vi "Begin.vi"(8 "error in":errorcluster) -> (0 "error out":errorcluster)   [LabVIEW 2015]
doc: "Called before other user functions, this VI is expected to open initial I/O refnums, load in file data, and do all program initialization. Notice that the <B>error out</B> terminal is simply used for data flow. Wiring it to other structures or subVIs ensures that this VI runs first."
uses:
  <vilib>/Rock Robotics/WPI/DriverStation/WPI_DriverStationRobotMode2.ctl
  Robot Global Data.vi
  <vilib>/Rock Robotics/WPI/Utilities/WPI_GetSetVariantRefNum.vi
  Library/REV Digit MXP/LabVIEW/REV Robotics Digit - Library.llb/REVDigit.lvlib
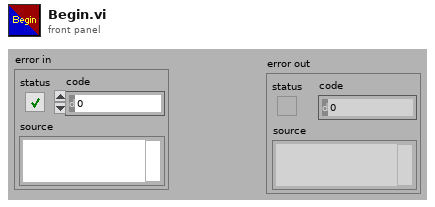
[diagram p1: front panel]
types:
  T1 = typedef "WPI_DriverStationRobotMode2.ctl" = enum16{"Autonomous Disabled", "Autonomous Enabled", "Teleop Disabled", "Teleop Enabled", "Disconnected", "Finish", "Test Disabled", "Test Enabled", "Emergency Stopped"}
  T2 = typedef "WPI_CompressorDevRef.ctl" = cluster{"DevStatus":errorcluster, "Pneumatics Control Module":u8}
  T3 = typedef "REVDigit.lvlib/REVDigitDefRef.ctl" = cluster{"HT16K33":T4, "Potentiometer":T6, "Button A":T8, "Button B":T8}
  T4 = typedef "WPI_I2CDevRef.ctl" = cluster{"DevStatus":errorcluster, "Device Address":u8, "Handle":i32, "I2C Bus":T5}
  T5 = typedef "i2c_bus.ctl" = enum16{"I2C On-Board", "I2C MXP", "Invalid"}
  T6 = typedef "WPI_AnalogChannelDevRef.ctl" = cluster{"DevStatus":errorcluster, "Analog Channel":T7}
  T7 = typedef "FPGA_AIChannel.ctl" = enum8{"AI 0", "AI 1", "AI 2", "AI 3", "AI MXP 0", "AI MXP 1", "AI MXP 2", "AI MXP 3", "Invalid"}
  T8 = typedef "WPI_DigitalInputDevRef.ctl" = cluster{"DevStatus":errorcluster, "DIO Channel":T9}
  T9 = typedef "FPGA_DIOChannel.ctl" = enum8{"DIO 0", "DIO 1", "DIO 2", "DIO 3", "DIO 4", "DIO 5", "DIO 6", "DIO 7", "DIO 8", "DIO 9", "DIO MXP 0", "DIO MXP 1", "DIO MXP 2", "DIO MXP 3", "DIO MXP 4", "DIO MXP 5", "DIO MXP 6", "DIO MXP 7", "DIO MXP 8", "DIO MXP 9", "DIO MXP 10", "DIO MXP 11", "DIO MXP 12", "DIO MXP 13", "DIO MXP 14", "DIO MXP 15", "Invalid"}
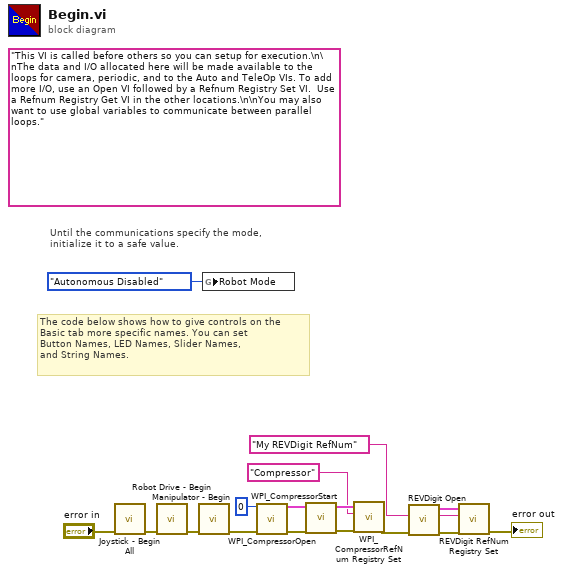
[diagram p0: block diagram]
diagram:
  (unwired) "This VI is called before others so you can setup for execution.\n\nThe data and I/O allocated here will be made available to the loops for camera, periodic, and to the Auto and TeleOp VIs. To add more I/O, use an Open VI followed by a Refnum Registry Set VI.  Use a Refnum Registry Get VI in the other locations.\n\nYou may also want to use global variables to communicate between parallel loops."
  # "The code below shows how to give controls on the\nBasic tab more specific names. You can set\nButton Names, LED Names, Slider Names,\nand String Names."
  # "Until the communications specify the mode,\ninitialize it to a safe value."
  n1 = call "Joystick - Begin All.vi"("error in (no error)"="error in") -> ("error out"=w15:errorcluster)  [unwired: 10 in]
  n2 = call "Robot Drive - Begin.vi"("error in (no error)"=w15) -> ("error out"=w14:errorcluster)  [unwired: 10 in]
  n3 = call "Manipulator - Begin.vi"("error in (no error)"=w14) -> ("error out"=w8:errorcluster)  [unwired: 10 in]
  n4 = global write "Robot Global Data.vi" "Robot Mode"(WPI_DriverStationRobotMode2."Autonomous Disabled" ("Robot Mode")) -> ()
  n5 = call <vilib>:"WPI_CompressorOpen.vi"("Pneumatics Control Module (0)"=u8 0, "error in (no error)"=w8) -> ("CompressorDevRef"=w9:T2, "error out"=w10:errorcluster)  [unwired: 12 in]
  n6 = call <vilib>:"WPI_CompressorStart.vi"("error in (no error)"=w10, "CompressorDevRef"=w9) -> ("error out"=w12:errorcluster, "CompressorDevRef"=w11:T2)  [unwired: 8 in]
  n7 = call <vilib>:"WPI_CompressorRefNum Registry Set.vi"("error in (no error)"=w12, "refnum name"="Compressor", "CompressorDevRef"=w11) -> ("error out"=w5:errorcluster)  [unwired: 7 in, 1 out]
  n8 = call "REVDigit Open.vi"("error in (no error)"=w5) -> ("error out"=w4:errorcluster, "REVDigitDefRef"=w3:T3)  [unwired: 9 in]
  n9 = call "REVDigit RefNum Registry Set.vi"("error in (no error)"=w4, "refnum name"="My REVDigit RefNum", "REVDigitRef"=w3) -> ("error out"=→"error out":errorcluster)  [unwired: 7 in, 1 out]
